vi "Run_4_Cmds.vi"(2 "USB DAQ Address":i32 format="%x") -> ()   [LabVIEW 2011]
panel:
  out "ACK 4":string
  out "Results 4":string
  out "ACK 3":string
  out "Results 3":string
  out "ACK 2":string
  out "Results 2":string
  out "ACK 1":string
  out "Results 1":string
  in  "Run Command 4":bool
  in  "Command 4":string
  in  "Run Command 3":bool
  in  "Command 3":string
  in  "Run Command 2":bool
  in  "Command 2":string
  in  "Run Command 1":bool
  in  "Command 1":string
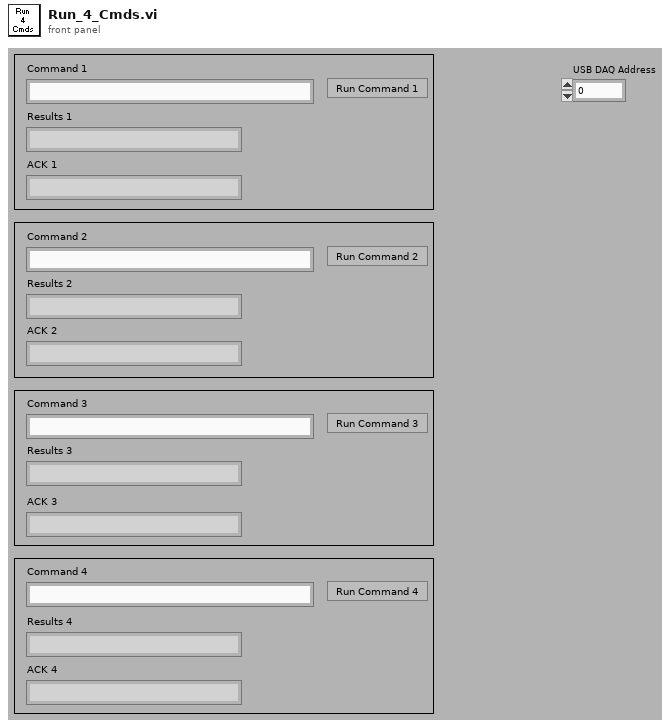
[diagram p1: front panel]
types:
  T1 = enum32{"Invalid", "Standard", "Closed", "Hidden", "Minimized", "Maximized"}
  T2 = enum16{"Always On", "Always Off", "Off While Running"}
  T3 = enum32{"invalid app kind", "Development System", "Run Time System", "Student Edition", "Embedded LabVIEW", "Evaluation", "Custom"}
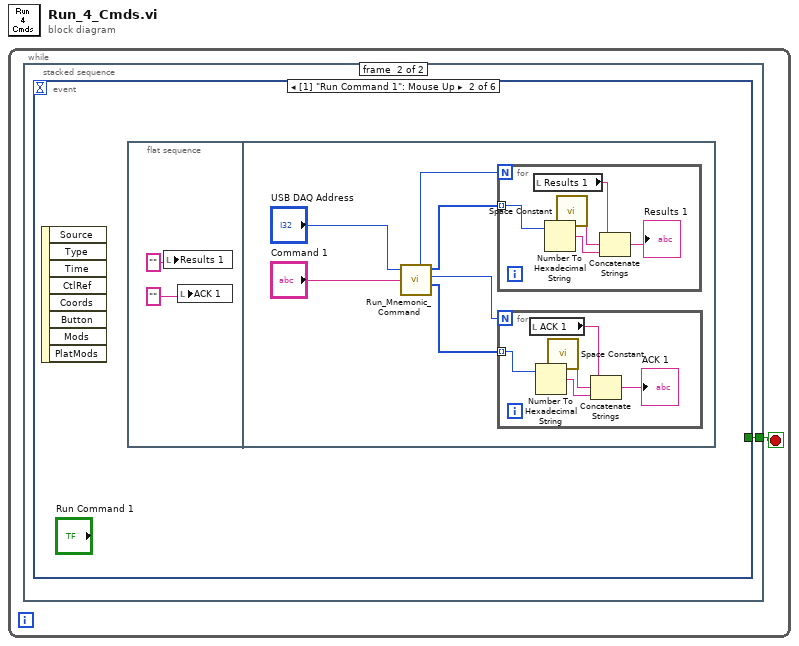
[diagram p0: block diagram]
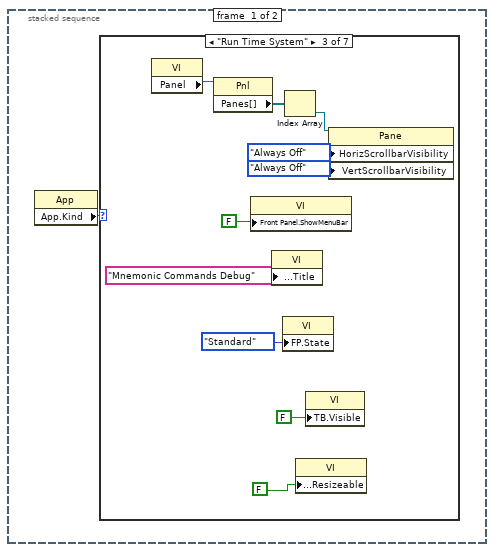
[diagram p2: hidden frame]
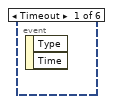
[diagram p9: hidden frame]
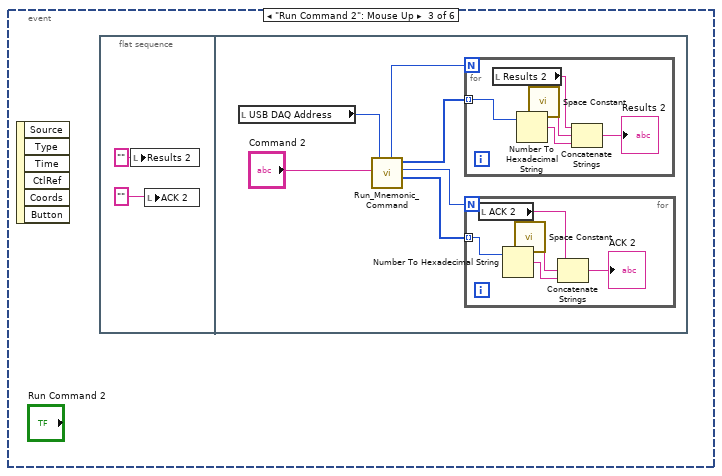
[diagram p10: hidden frame]
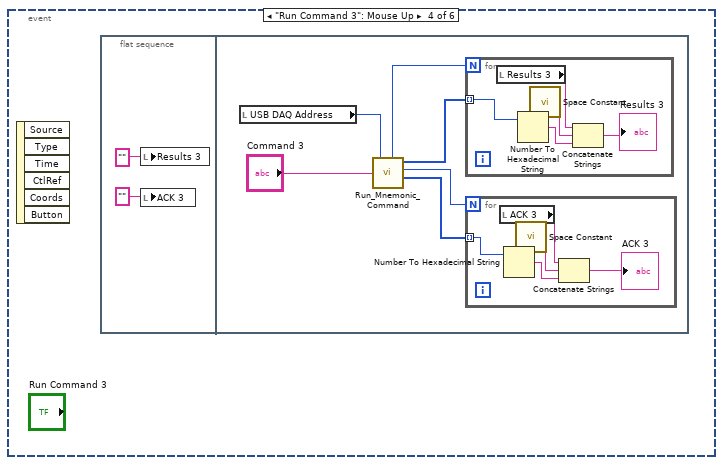
[diagram p11: hidden frame]
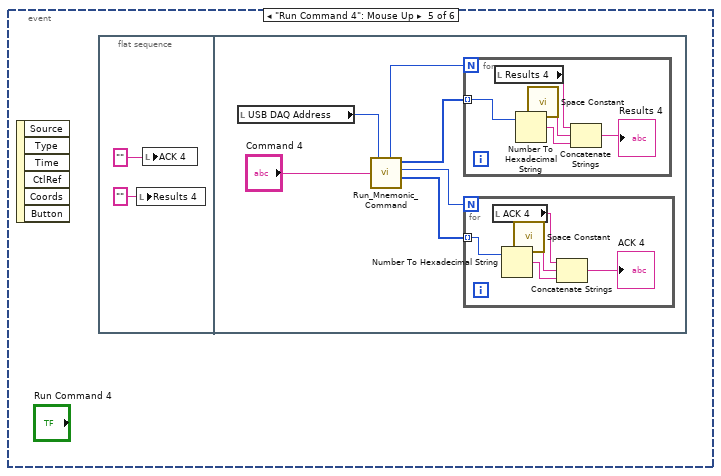
[diagram p12: hidden frame]
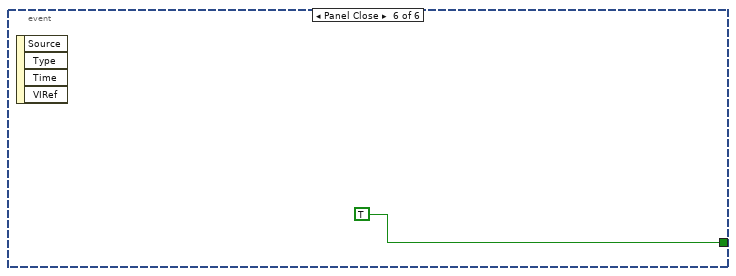
[diagram p13: hidden frame]
diagram:
  n1 = while {
    stop <- w1 stop-if-true
    n2 = stacked-sequence {
      tunnel: [_ w13] -> w1
      frame #0 {
        n3 = property class="App"() -> ("App.Kind"=w2:T3)  [unwired: 2 in, 2 out]
        n4 = case shown="\"Run Time System\"" w2 {
          frame "invalid app kind", Default {
          }
          frame "Development System" {
          }
          frame "Run Time System" {
            n5 = property class="VI"() -> ("Panel"=w12:refnum<vi>)  [unwired: 2 in, 2 out]
            n6 = property class="Pnl"(reference=w12) -> ("Panes[]"=w11:refnum<vi>[])  [unwired: 1 in, 2 out]
            n7 = property class="VI"("Front Panel.ShowMenuBar"=FALSE ("Front Panel Window:Show Menu Bar")) -> ()  [unwired: 2 in, 2 out]
            n8 = property class="VI"("Front Panel.Title"="Mnemonic Commands Debug" ("Front Panel Window:Title")) -> ()  [unwired: 2 in, 2 out]
            n9 = property class="VI"("FP.State"=T1."Standard" ("Front Panel Window:State")) -> ()  [unwired: 2 in, 2 out]
            n10 = Index Array(array=w11) -> (element=w10:refnum<vi>)  [unwired: 1 in]
            n11 = property class="VI"("Front Panel.Resizeable"=FALSE ("Front Panel Window:Resizeable")) -> ()  [unwired: 2 in, 2 out]
            n12 = property class="VI"("TB.Visible"=FALSE ("Front Panel Window:Resizeable")) -> ()  [unwired: 2 in, 2 out]
            n13 = property class="Pane"(reference=w10, "HorizScrollbarVisibility"=T2."Always Off" ("Horizontal Scrollbar Visibility"), "VertScrollbarVisibility"=T2."Always Off" ("Vertical Scrollbar Visibility")) -> ()  [unwired: 1 in, 2 out]
          }
          frame "Student Edition" {
          }
          frame "Embedded LabVIEW" {
          }
          frame "Evaluation" {
          }
          frame "Custom" {
          }
        }
      }
      frame #1 {
        n14 = event shown="[1] \"Run Command 1\": Mouse Up" {
          selector: _ -> [_ _ _ _ _ _]
          dyn-events: _ -> [_ _ _ _ _ _]
          timeout: _ -> [_ _ _ _ _ _]
          tunnel: [_ _ _ _ _ TRUE] -> w13
          event Timeout {
            n15 = event-data() -> ()  [unwired: 1 in, 2 out]
          }
          event "Run Command 1": Mouse Up {
            n16 = event-data() -> ()  [unwired: 1 in, 8 out]
            n17 = flat-sequence {
              frame #0 {
                n18 = local write "Results 1"("" ("Results 1")) -> ()
                n19 = local write "ACK 1"("" ("Results 1")) -> ()
              }
              frame #1 {
                n20 = call "Run_Mnemonic_Command.vi"("command string"="Command 1", "Device address"="USB DAQ Address") -> ("ACKS-array"=w16:u8[], "ACKS count"=w17:i32, "result count"=w18:i32, "result-array"=w19:u8[])  [unwired: 2 in, 1 out]
                n21 = for {
                  N: w18 -> [_]
                  tunnel: w19 -> [w31] mode=indexing
                  n22 = local read "Results 1"() -> (w30:string)
                  n23 = Number To Hexadecimal String(2:w31) -> (0:w27:string)  [unwired: 1 in]
                  n24 = call <vilib>:"Space Constant.vi"() -> ("String"=w28:string)
                  n25 = Concatenate Strings(w30, w28, w27) -> (→"Results 1":string)
                }
                n26 = for {
                  N: w17 -> [_]
                  tunnel: w16 -> [w26] mode=indexing
                  n27 = local read "ACK 1"() -> (w22:string)
                  n28 = Number To Hexadecimal String(2:w26) -> (0:w24:string)  [unwired: 1 in]
                  n29 = call <vilib>:"Space Constant.vi"() -> ("String"=w25:string)
                  n30 = Concatenate Strings(w22, w25, w24) -> (→"ACK 1":string)
                }
              }
            }
          }
          event "Run Command 2": Mouse Up {
            n31 = event-data() -> ()  [unwired: 1 in, 6 out]
            n32 = flat-sequence {
              frame #0 {
                n33 = local write "Results 2"("" ("Results 1")) -> ()
                n34 = local write "ACK 2"("" ("Results 1")) -> ()
              }
              frame #1 {
                n35 = local read "USB DAQ Address"() -> (w34:i32)
                n36 = call "Run_Mnemonic_Command.vi"("command string"="Command 2", "Device address"=w34) -> ("ACKS-array"=w36:u8[], "ACKS count"=w37:i32, "result count"=w38:i32, "result-array"=w39:u8[])  [unwired: 2 in, 1 out]
                n37 = for {
                  N: w38 -> [_]
                  tunnel: w39 -> [w49] mode=indexing
                  n38 = local read "Results 2"() -> (w46:string)
                  n39 = Number To Hexadecimal String(2:w49) -> (0:w47:string)  [unwired: 1 in]
                  n40 = call <vilib>:"Space Constant.vi"() -> ("String"=w48:string)
                  n41 = Concatenate Strings(w46, w48, w47) -> (→"Results 2":string)
                }
                n42 = for {
                  N: w37 -> [_]
                  tunnel: w36 -> [w44] mode=indexing
                  n43 = local read "ACK 2"() -> (w41:string)
                  n44 = Number To Hexadecimal String(2:w44) -> (0:w42:string)  [unwired: 1 in]
                  n45 = call <vilib>:"Space Constant.vi"() -> ("String"=w43:string)
                  n46 = Concatenate Strings(w41, w43, w42) -> (→"ACK 2":string)
                }
              }
            }
          }
          event "Run Command 3": Mouse Up {
            n47 = event-data() -> ()  [unwired: 1 in, 6 out]
            n48 = flat-sequence {
              frame #0 {
                n49 = local write "Results 3"("" ("Results 1")) -> ()
                n50 = local write "ACK 3"("" ("Results 1")) -> ()
              }
              frame #1 {
                n51 = local read "USB DAQ Address"() -> (w53:i32)
                n52 = call "Run_Mnemonic_Command.vi"("command string"="Command 3", "Device address"=w53) -> ("ACKS-array"=w54:u8[], "ACKS count"=w55:i32, "result count"=w56:i32, "result-array"=w57:u8[])  [unwired: 2 in, 1 out]
                n53 = for {
                  N: w56 -> [_]
                  tunnel: w57 -> [w67] mode=indexing
                  n54 = local read "Results 3"() -> (w64:string)
                  n55 = Number To Hexadecimal String(2:w67) -> (0:w65:string)  [unwired: 1 in]
                  n56 = call <vilib>:"Space Constant.vi"() -> ("String"=w66:string)
                  n57 = Concatenate Strings(w64, w66, w65) -> (→"Results 3":string)
                }
                n58 = for {
                  N: w55 -> [_]
                  tunnel: w54 -> [w62] mode=indexing
                  n59 = local read "ACK 3"() -> (w59:string)
                  n60 = Number To Hexadecimal String(2:w62) -> (0:w60:string)  [unwired: 1 in]
                  n61 = call <vilib>:"Space Constant.vi"() -> ("String"=w61:string)
                  n62 = Concatenate Strings(w59, w61, w60) -> (→"ACK 3":string)
                }
              }
            }
          }
          event "Run Command 4": Mouse Up {
            n63 = event-data() -> ()  [unwired: 1 in, 6 out]
            n64 = flat-sequence {
              frame #0 {
                n65 = local write "Results 4"("" ("Results 1")) -> ()
                n66 = local write "ACK 4"("" ("Results 1")) -> ()
              }
              frame #1 {
                n67 = local read "USB DAQ Address"() -> (w71:i32)
                n68 = call "Run_Mnemonic_Command.vi"("command string"="Command 4", "Device address"=w71) -> ("ACKS-array"=w72:u8[], "ACKS count"=w73:i32, "result count"=w74:i32, "result-array"=w75:u8[])  [unwired: 2 in, 1 out]
                n69 = for {
                  N: w74 -> [_]
                  tunnel: w75 -> [w85] mode=indexing
                  n70 = local read "Results 4"() -> (w82:string)
                  n71 = Number To Hexadecimal String(2:w85) -> (0:w83:string)  [unwired: 1 in]
                  n72 = call <vilib>:"Space Constant.vi"() -> ("String"=w84:string)
                  n73 = Concatenate Strings(w82, w84, w83) -> (→"Results 4":string)
                }
                n74 = for {
                  N: w73 -> [_]
                  tunnel: w72 -> [w80] mode=indexing
                  n75 = local read "ACK 4"() -> (w77:string)
                  n76 = Number To Hexadecimal String(2:w80) -> (0:w78:string)  [unwired: 1 in]
                  n77 = call <vilib>:"Space Constant.vi"() -> ("String"=w79:string)
                  n78 = Concatenate Strings(w77, w79, w78) -> (→"ACK 4":string)
                }
              }
            }
          }
          event Panel Close {
            n79 = event-data() -> ()  [unwired: 1 in, 4 out]
          }
        }
      }
    }
  }
